vi "Get Server gRPC UEs.vi"(11 "OOP Server in":refnum<class "NW and PSD_server.lvclass">) -> (2 "Server RPC Methods":T1, 3 "OOP Server out":refnum<class "NW and PSD_server.lvclass">)   [LabVIEW 2019, in "NW and PSD_server.lvlib" / "NW and PSD_server.lvclass"]
uses:
  NW and PSD_server.lvclass
  typeDefs/Server gRPC UEs.ctl
  <vilib>/gRPC/LabVIEW gRPC Library/Server API/typeDefs/gRPCId Cluster.ctl
  <vilib>/gRPC/LabVIEW gRPC Library/Server API/typeDefs/grpcId.ctl
  NW and PSD_server.lvclass/NW and PSD_server.ctl
  <vilib>/gRPC/LabVIEW gRPC Library/gprc-lvsupport-release.lvlib
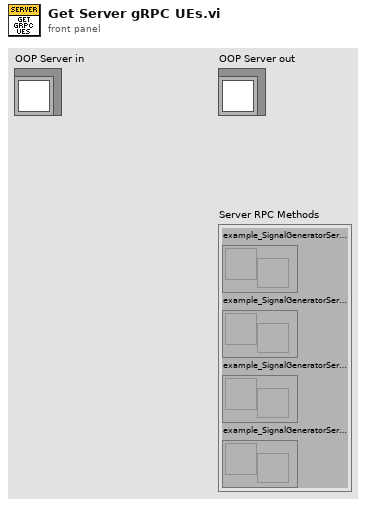
[diagram p1: front panel]
types:
  T1 = typedef "NW and PSD_server.lvlib/NW and PSD_server.lvclass/Server gRPC UEs.ctl" = cluster{"example_SignalGeneratorService_ApplySignalParameters gRPC UE":refnum<user-event>, "example_SignalGeneratorService_ApplyNoiseParameters gRPC UE":refnum<user-event>, "example_SignalGeneratorService_GenerateSignal gRPC UE":refnum<user-event>, "example_SignalGeneratorService_GetAnalyzedParameters gRPC UE":refnum<user-event>}
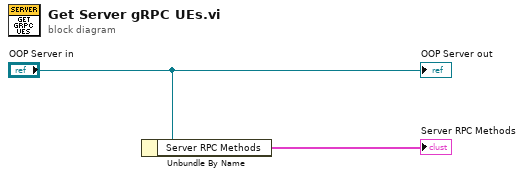
[diagram p0: block diagram]
diagram:
  n1 = Unbundle By Name("OOP Server in") -> ("Server RPC Methods"=→"Server RPC Methods":T1)
  "OOP Server out" <- "OOP Server in"
